vi "Monitoring.vi"(4 "Channels":string="N2,N6,E2,E6,S2,S6,W2,W6", 5 "MessageQueues":T1, 6 "Recorded Channels":i32=8, 7 "task in":refnum<k21>, 9 "Gain (V/nA)":dbl=-0.45, 10 "No. of Samples / Loop":i64=1000, 11 "tdms file out":refnum<k34>) -> (0 "error out":errorcluster)   [LabVIEW 2024]
uses:
  MessageQueues.ctl
  <vilib>/httpClient/ClientHandle.ctl
  <vilib>/DAQmx/read.llb/DAQmx Read (Analog 1D Wfm NChan NSamp).vi
  <vilib>/DAQmx/miscellaneous.llb/DAQmx Fill In Error Info.vi
  <vilib>/httpClient/LabVIEWHTTPClient.lvlib
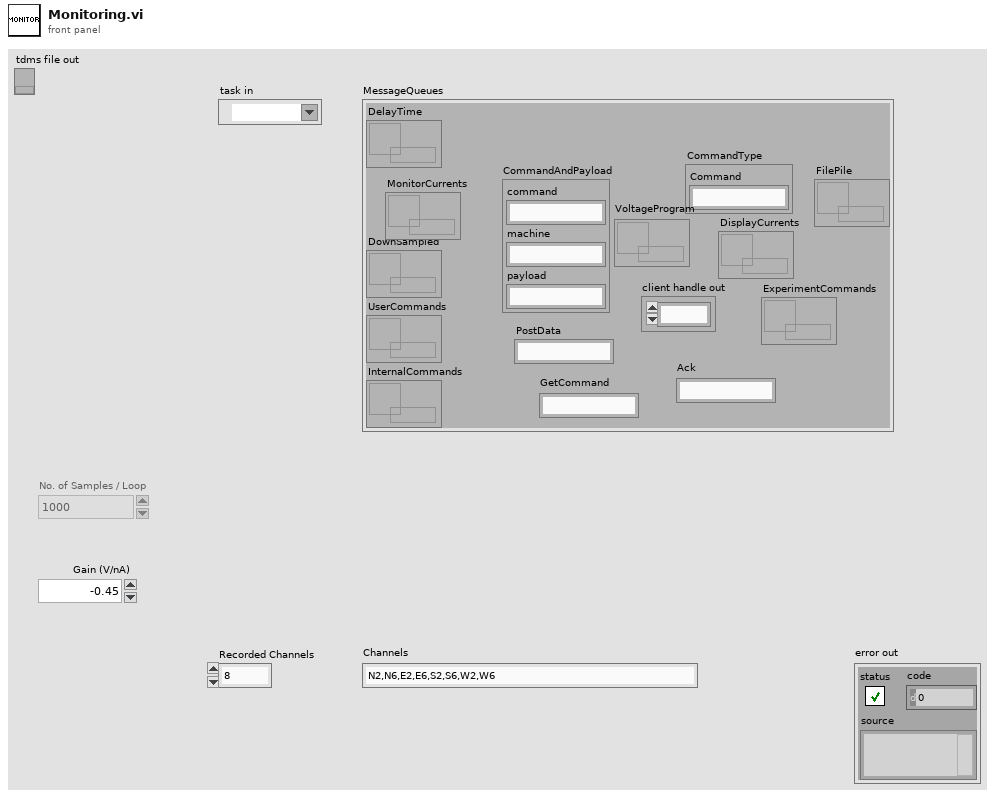
[diagram p1: front panel]
types:
  T1 = typedef "MessageQueues.ctl" = cluster{"DelayTime":refnum<queue>, "DownSampled":refnum<queue>, "UserCommands":refnum<queue>, "InternalCommands":refnum<queue>, "CommandType":cluster{"Command":string}, "CommandAndPayload":cluster{"command":string, "machine":string, "payload":string}, "client handle out":T2, "PostData":string, "GetCommand":string, "Ack":string, "VoltageProgram":refnum<queue>, "ExperimentCommands":refnum<queue>, "DisplayCurrents":refnum<queue>, "MonitorCurrents":refnum<queue>, "FilePile":refnum<queue>}
  T2 = typedef "LabVIEWHTTPClient.lvlib/ClientHandle.ctl" = refnum<k1>
  T3 = cluster{"Waveforms":waveform(dbl)[], "file":refnum<k34>}
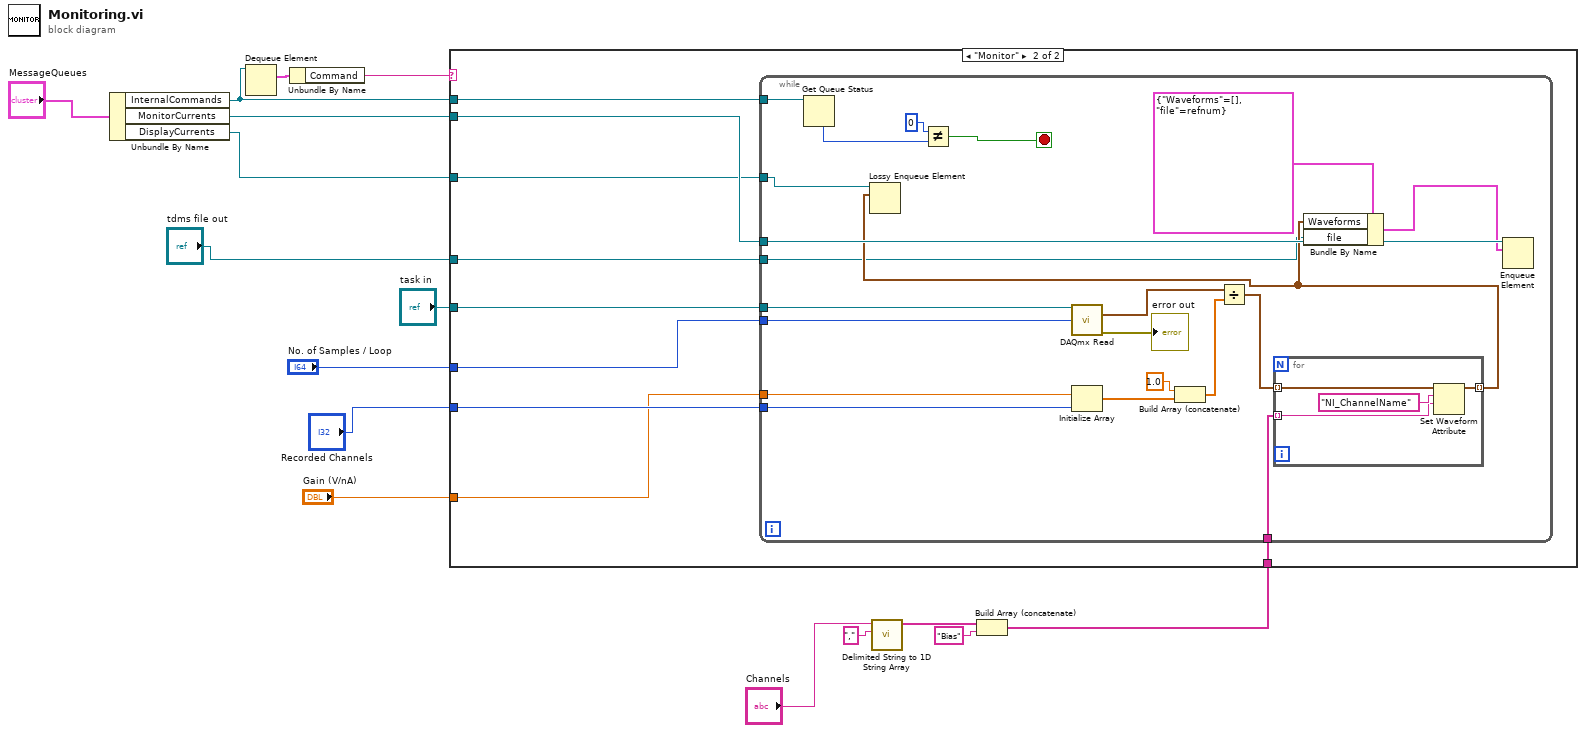
[diagram p0: block diagram]
diagram:
  n1 = Unbundle By Name("MessageQueues") -> ("InternalCommands"=w16:refnum<queue>, "MonitorCurrents"=w11:refnum<queue>, "DisplayCurrents"=w2:refnum<queue>)
  n2 = Dequeue Element(queue=w16) -> (element=w13:cluster{"Command":string})  [unwired: 2 in, 3 out]
  n3 = Unbundle By Name(w13) -> ("Command"=w14:string)
  n4 = call <vilib>:"Delimited String to 1D String Array.vi"("delimiter"="," ("search string/char (-)"), "delimited string"="Channels") -> ("string array"=w7:string[])  [unwired: 9 in]
  n5 = Build Array (concatenate)(w7, "Bias") -> (w3:string[])
  n6 = case shown="\"Monitor\"" w14 {
    tunnel: "task in" -> [_ w25]
    tunnel: w16 -> [_ w24]
    tunnel: w11 -> [_ w23]
    tunnel: "Recorded Channels" -> [_ w22]
    tunnel: "No. of Samples / Loop" -> [_ w21]
    tunnel: "Gain (V/nA)" -> [_ w20]
    tunnel: w3 -> [_ w19]
    tunnel: w2 -> [_ w18]
    tunnel: "tdms file out" -> [_ w17]
    frame "False", Default {
    }
    frame "Monitor" {
      n7 = while {
        tunnel: w23 -> [w42]
        tunnel: w25 -> [w40]
        tunnel: w24 -> [w39]
        tunnel: w22 -> [w34]
        tunnel: w21 -> [w33]
        tunnel: w20 -> [w32]
        tunnel: w19 -> [w31]
        tunnel: w18 -> [w30]
        tunnel: w17 -> [w26]
        stop <- w35 stop-if-true
        n8 = Get Queue Status(queue=w39) -> (# elements in queue=w38:i32)  [unwired: 2 in, 7 out]
        n9 = Not Equal?(x=0, y=w38) -> (x != y?=w35:bool)
        n10 = call-poly <vilib>:"DAQmx Read.vi"("task/channels in"=w40, "number of samples per channel"=w33) -> ("data"=w43:waveform(dbl)[], "error out"=→"error out":errorcluster)  [unwired: 11 in, 1 out]
        n11 = Initialize Array(w32, w34) -> (w46:dbl[])
        n12 = Build Array (concatenate)(1.0 ("Gain (V/nA)"), w46) -> (w44:dbl[])
        n13 = Divide(x=w43, y=w44) -> (x/y=w41:waveform(dbl)[])
        n14 = for {
          tunnel: w41 -> [w50] mode=indexing
          tunnel: w31 -> [w48] mode=indexing
          tunnel: [w47] -> w28 mode=indexing
          n15 = Set Waveform Attribute(5:w48, 6:"NI_ChannelName" ("name"), 7:w50) -> (3:w47:waveform(dbl))  [unwired: 1 in, 2 out]
        }
        n16 = Lossy Enqueue Element(queue=w30, element=w28) -> ()  [unwired: 1 in, 4 out]
        n17 = Bundle By Name(cluster=T3 {"Waveforms"=[], "file"=refnum} ("element"), "Waveforms"=w28, "file"=w26) -> (w27:T3)
        n18 = Enqueue Element(queue=w42, element=w27) -> ()  [unwired: 2 in, 3 out]
      }
    }
  }
